vi "main.vi"() -> ()   [LabVIEW 2024]
uses:
  <vilib>/FPGAPlugInAG/NI 9147/niLvFpga_Open_NI 9147.vi
  <vilib>/rvi/interface/common/dynamic/niFpgaDynamicAddResources.vi
  <vilib>/FPGAPlugInAG/Dynamic/niLvFpga_Run_Dynamic.vi
  <vilib>/FPGAPlugInAG/Dynamic/niLvFpga_Close_Dynamic.vi
  <vilib>/rvi/interface/nirviOpenFPGA/nirviOpenFPGA.xnode
  FPGA Bitfiles/dircdaq-automate_FPGATarget_fpga_RyAY8MzD2n8.lvbitx
  fpga.vi
  <vilib>/rvi/interface/nirviMethod/nirviMethod.xnode
  <vilib>/rvi/interface/nirviCloseFPGA/nirviCloseFPGA.xnode
panel:
  out "fpga-ref":refnum<k20>
  out "all data":dbl[](array[numeric])
  out "pd3/pd1":dbl
  out "prog-heartbeat":bool
  in  "get-meas":bool
  in  "stop":bool
  # "pd1 avg"
  # "pd2 avg"
  # "pd3 avg"
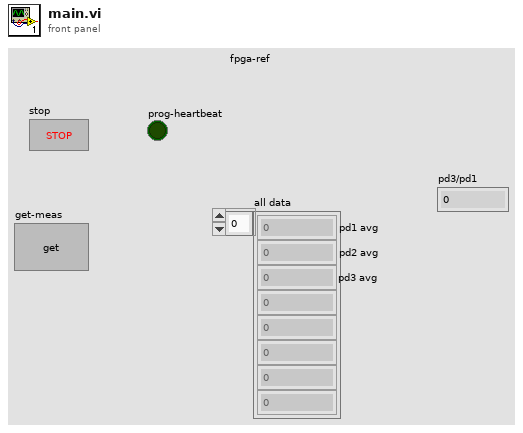
[diagram p1: front panel]
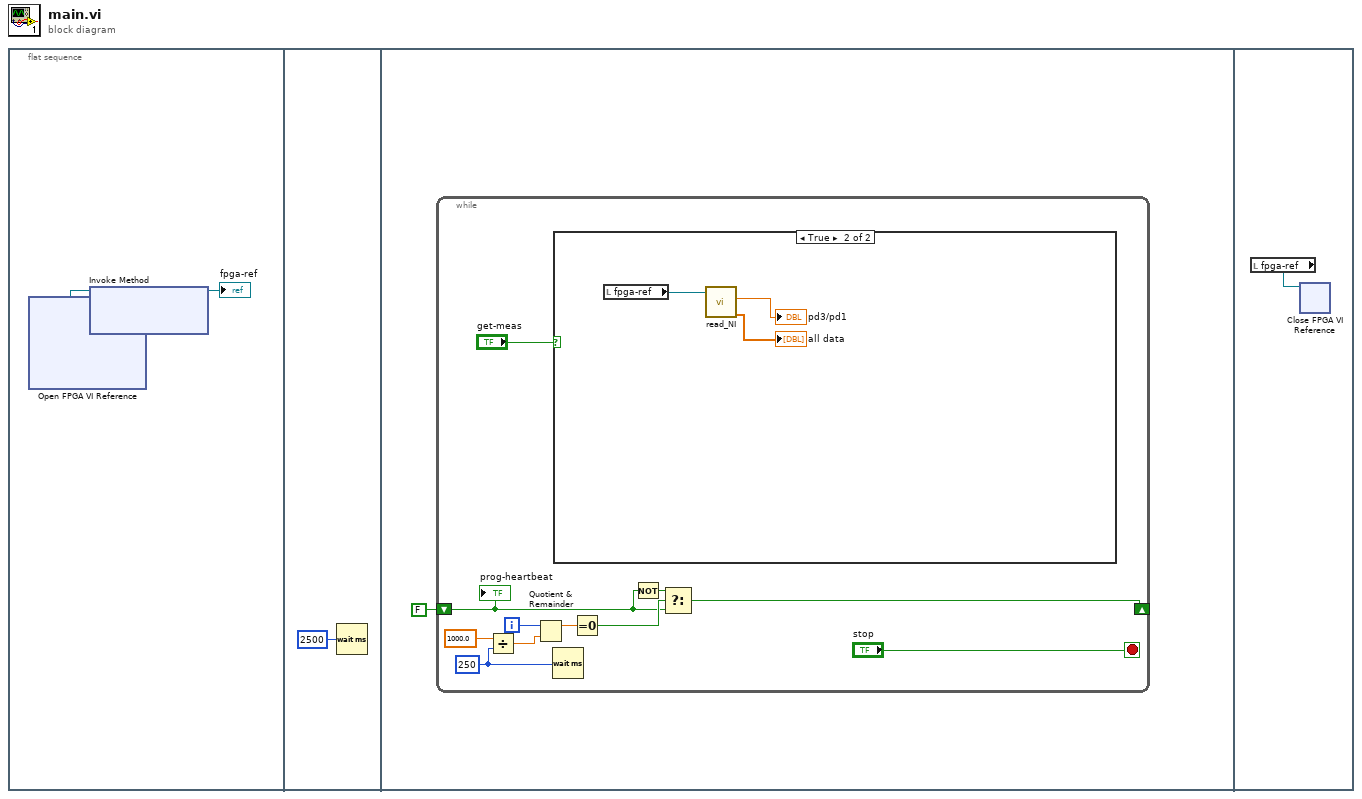
[diagram p0: block diagram]
diagram:
  n1 = flat-sequence {
    frame #0 {
      n2 = xnode "Open FPGA VI Reference"() -> ("FPGA VI Reference Out"=w2:refnum<k20>)  [unwired: 2 in, 1 out]
      n3 = xnode "Invoke Method"("FPGA VI Reference In"=w2) -> ("FPGA VI Reference Out"=→"fpga-ref":refnum<k20>)  [unwired: 2 in, 1 out]
    }
    frame #1 {
      n4 = Wait (ms)(milliseconds to wait=u32 2500) -> ()  [unwired: 1 out]
    }
    frame #2 {
      n5 = while {
        shift-right: [w10] -> _
        shift-left: FALSE -> [w8]
        i -> [w13]
        stop <- "stop" stop-if-true
        w5 = u32 250 ("milliseconds to wait")
        n6 = Divide(x=1000.0, y=w5) -> (x/y=w7:dbl)
        n7 = Quotient & Remainder(x=w13, y=w7) -> (x-y*floor(x/y)=w12:dbl)  [unwired: 1 out]
        n8 = Wait (ms)(milliseconds to wait=w5) -> ()  [unwired: 1 out]
        n9 = case shown="True" "get-meas" {
          frame False {
          }
          frame True {
            n10 = local read "fpga-ref"() -> (w16:refnum<k20>)
            n11 = call "read_NI.vi"("fpga-ref-in"=w16) -> ("all_pds"=→"all data":dbl[], "pd3/pd1"=→"pd3/pd1":dbl)  [unwired: 7 in, 2 out]
          }
        }
        n12 = Equal To 0?(x=w12) -> (x = 0?=w11:bool)
        n13 = Not(x=w8) -> (.not. x?=w9:bool)
        n14 = Select(t=w9, s=w11, f=w8) -> (s? t:f=w10:bool)
        "prog-heartbeat" <- w8
      }
    }
    frame #3 {
      n15 = local read "fpga-ref"() -> (w19:refnum<k20>)
      n16 = xnode "Close FPGA VI Reference"("FPGA VI Reference In"=w19) -> ()  [unwired: 1 in, 1 out]
    }
  }
